vi "PathPlanner_GridPosition_Print.vi"(11 "GridPosition":T1) -> (3 "Position String":string)   [LabVIEW 2019, in "PathPlanner24.lvlib"]
uses:
  TypeDef/PathPlannerFinderGridPosition.ctl
  PathPlanner24.lvlib
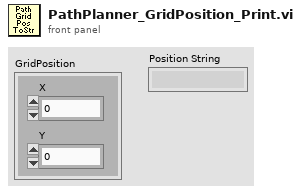
[diagram p1: front panel]
types:
  T1 = typedef "PathPlanner24.lvlib/PathPlannerFinderGridPosition.ctl" = cluster{"X":i32, "Y":i32}
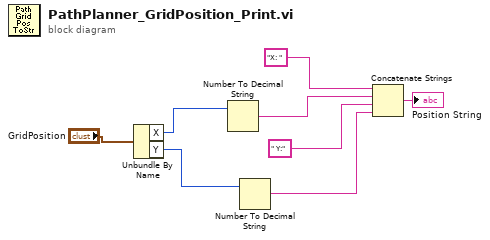
[diagram p0: block diagram]
diagram:
  n1 = Unbundle By Name("GridPosition") -> ("X"=w7:i32, "Y"=w6:i32)
  n2 = Number To Decimal String(number=w7) -> (decimal integer string=w4:string)  [unwired: 1 in]
  n3 = Number To Decimal String(number=w6) -> (decimal integer string=w2:string)  [unwired: 1 in]
  n4 = Concatenate Strings("X: " ("string"), w4, " Y:" ("string"), w2) -> (→"Position String":string)
